vi "Shutdown Core.vi"(8 "error in (no error)":errorcluster, 11 "SLSC Switch Consumer in":refnum<class "SLSC Switch Consumer.lvclass">) -> (0 "error out":errorcluster, 3 "SLSC Switch Consumer out":refnum<class "SLSC Switch Consumer.lvclass">)   [LabVIEW 2017, in "SLSC Switch Messaging.lvlib" / "SLSC Switch Consumer.lvclass"]
uses:
  SLSC Switch Consumer.lvclass
  SLSC Switch Consumer.lvclass/SLSC Switch Consumer.ctl
  <vilib>/userdefined/High Color/SLSC_Switch/nislscslSession.ctl
  <vilib>/SLSC_Switch/SLSC Switch.lvlib
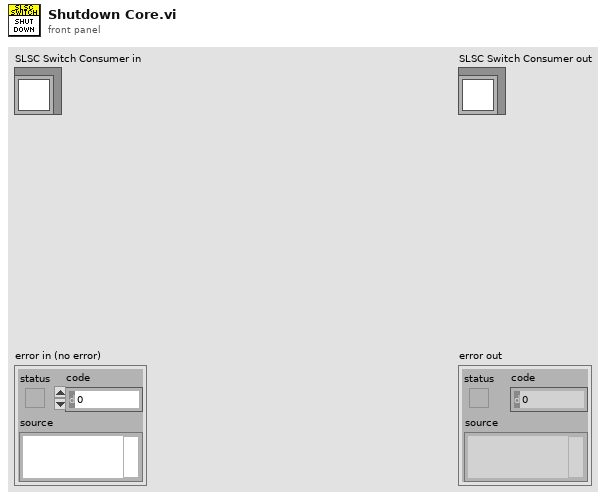
[diagram p1: front panel]
types:
  T1 = typedef "nislscslSession.ctl" = refnum<k20>
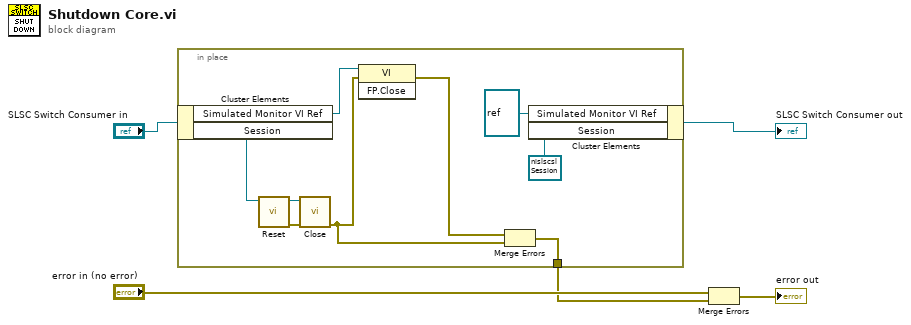
[diagram p0: block diagram]
diagram:
  n1 = in-place {
    in-place-border: [w6] -> w3
    n2 = in-place-cluster #1("SLSC Switch Consumer in") -> ("Simulated Monitor VI Ref"=w10:refnum<vi>, "Session"=w14:T1)
    n3 = call <vilib>:"Reset.vi"("session in"=w14) -> ("error out"=w11:errorcluster, "session out"=w12:T1)  [unwired: 9 in]
    n4 = call <vilib>:"Close.vi"("error in (no error)"=w11, "session in"=w12) -> ("error out"=w7:errorcluster)  [unwired: 9 in]
    n5 = invoke class="VI" method="FP.Close"(reference=w10, error in=w7) -> (error out=w8:errorcluster)  [unwired: 1 in, 2 out]
    n6 = Merge Errors(w8, w7) -> (w6:errorcluster)
    n7 = in-place-cluster #1("Simulated Monitor VI Ref"=refnum<vi> refnum, "Session"=T1 refnum) -> (→"SLSC Switch Consumer out":refnum<class "SLSC Switch Consumer.lvclass">)
  }
  n8 = Merge Errors("error in (no error)", w3) -> (→"error out":errorcluster)
